vi "Stabilize.vi"(1 "Angle":dbl) -> (0 "result":dbl)   [LabVIEW 2011]
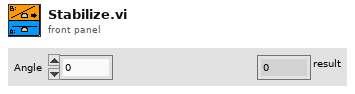
[diagram p1: front panel]
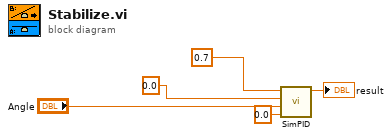
[diagram p0: block diagram]
diagram:
  n1 = call "SimPID.vi"("Range"=0.0, "Position"="Angle", "Set Point"=0.0, "Gain"=0.7) -> ("result"=→"result":dbl)  [unwired: 5 in, 1 out]
